vi "Setup.vi"(8 "error in (no error)":errorcluster caption="Fehler (Eingang, kein Fehler)", 11 "Moveo Eingang":refnum<class "Moveo.lvclass">) -> (0 "error out":errorcluster caption="Fehler (Ausgang)", 3 "Moveo Ausgang":refnum<class "Moveo.lvclass">)   [LabVIEW 2019, in "Moveo.lvclass"]
uses:
  Moveo.lvclass
  Moveo.lvclass/Moveo.ctl
  MoveoSerialClass/MoveoSerial.lvclass
panel:
  in  "VISA resource name":refnum<visa-resource-name>
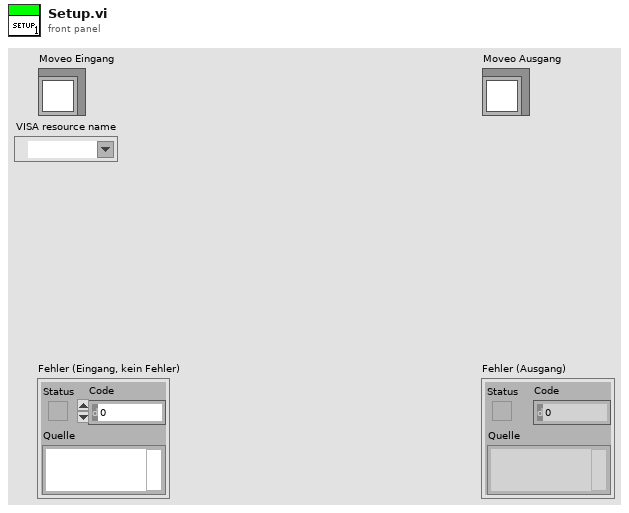
[diagram p1: front panel]
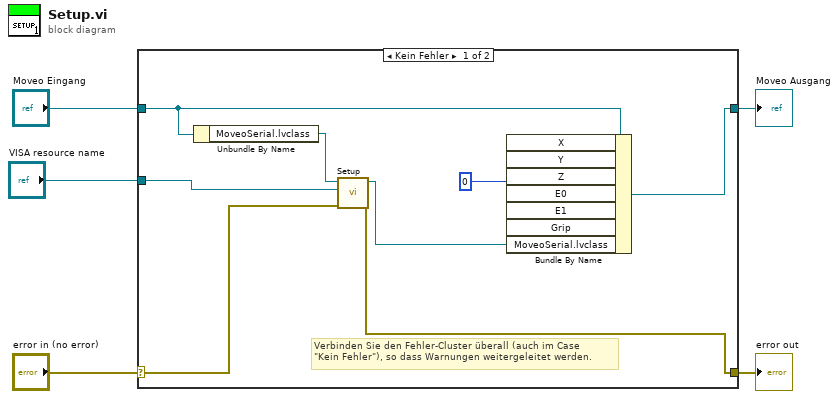
[diagram p0: block diagram]
diagram:
  n1 = case shown="Kein Fehler" "error in (no error)" {
    selector: "error in (no error)" -> [w8 w15]
    tunnel: [w6 w15] -> w4
    tunnel: [w13 w14] -> w2
    tunnel: "Moveo Eingang" -> [w11 w14]
    tunnel: "VISA resource name" -> [w9 _]
    frame No Error {
      w12 = i16 0 ("X")
      # "Verbinden Sie den Fehler-Cluster überall (auch im Case\n\"Kein Fehler\"), so dass Warnungen weitergeleitet werden."
      n2 = Unbundle By Name(w11) -> ("MoveoSerial.lvclass"=w10:refnum<class "MoveoSerial.lvclass">)
      n3 = call-dynamic "Setup.vi"("error in (no error)"=w8, "VISA resource name"=w9, "MoveoSerial Eingang"=w10) -> ("error out"=w6:errorcluster, "MoveoSerial Ausgang"=w7:refnum<class "MoveoSerial.lvclass">)  [unwired: 7 in]
      n4 = Bundle By Name(cluster=w11, "X"=w12, "Y"=w12, "Z"=w12, "E0"=w12, "E1"=w12, "Grip"=w12, "MoveoSerial.lvclass"=w7) -> (w13:refnum<class "Moveo.lvclass">)
    }
    frame Error {
    }
  }
  "error out" <- w4
  "Moveo Ausgang" <- w2
